vi "Xeryon convert statusbits.vi"(4 "single value out":i32) -> (1 "Cluster":T1)   [LabVIEW 2014]
uses:
  Xeryon status bits.ctl
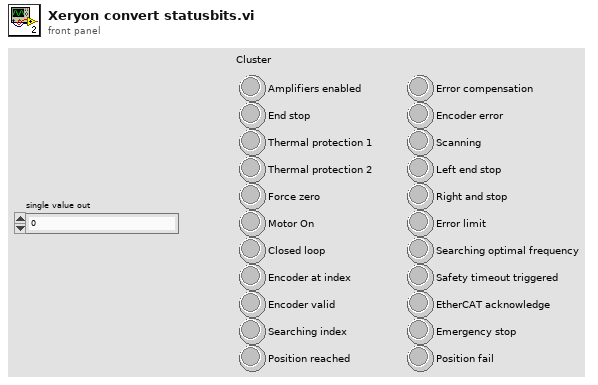
[diagram p1: front panel]
types:
  T1 = typedef "Xeryon status bits.ctl" = cluster{"Amplifiers enabled":bool, "End stop":bool, "Thermal protection 1":bool, "Thermal protection 2":bool, "Force zero":bool, "Motor On":bool, "Closed loop":bool, "Encoder at index":bool, "Encoder valid":bool, "Searching index":bool, "Position reached":bool, "Error compensation":bool, "Encoder error":bool, "Scanning":bool, "Left end stop":bool, "Right and stop":bool, "Error limit":bool, "Searching optimal frequency":bool, "Safety timeout triggered":bool, "EtherCAT acknowledge":bool, "Emergency stop":bool, "Position fail":bool}
  T2 = cluster{"Boolean array[0]":bool, "Boolean array[1]":bool, "Boolean array[2]":bool, "Boolean array[3]":bool, "Boolean array[4]":bool, "Boolean array[5]":bool, "Boolean array[6]":bool, "Boolean array[7]":bool, "Boolean array[8]":bool, "Boolean array[9]":bool, "Boolean array[10]":bool, "Boolean array[11]":bool, "Boolean array[12]":bool, "Boolean array[13]":bool, "Boolean array[14]":bool, "Boolean array[15]":bool, "Boolean array[16]":bool, "Boolean array[17]":bool, "Boolean array[18]":bool, "Boolean array[19]":bool, "Boolean array[20]":bool, "Boolean array[21]":bool}
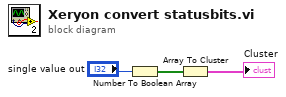
[diagram p0: block diagram]
diagram:
  n1 = Number To Boolean Array(number="single value out") -> (Boolean array=w2:bool[])
  n2 = Array To Cluster(array=w2) -> (cluster=→"Cluster":T2)
